vi "runtest update field value.vi"(1 "Process SPARTAN SN (F)":bool, 4 "ProcessNextItem? (f)":bool, 6 "User/Station":T1, 7 "POST (empty)":T4, 8 "error in (no error)":errorcluster, 9 "Model Number (\"\")":string, 10 "Field":T6={"ixField"=0, "iSequenceOrder"=0, "sxFieldId"="", "sxSequenceId"="", "sDisplayName"="", "sValue"="", "sUnits"="", "nDataType"=enum."timestamp", "nNextItem"=enum."Reset", "fSystem"=FALSE, "fSystemValue"=FALSE, "fRequired"=FALSE, "fSetAtTest"=FALSE, "fTestField"=FALSE, "fDeleted"=FALSE, "fIndexed"=FALSE, "fFreeList"=FALSE}, 11 "Connection Refnum":T5) -> (0 "error out":errorcluster, 2 "updated Field":T6={"ixField"=0, "iSequenceOrder"=0, "sxFieldId"="", "sxSequenceId"="", "sDisplayName"="", "sValue"="", "sUnits"="", "nDataType"=enum."timestamp", "nNextItem"=enum."Reset", "fSystem"=FALSE, "fSystemValue"=FALSE, "fRequired"=FALSE, "fSetAtTest"=FALSE, "fTestField"=FALSE, "fDeleted"=FALSE, "fIndexed"=FALSE, "fFreeList"=FALSE}, 3 "Connection Refnum":T5, 5 "remaining POST":T4)   [LabVIEW 2011]
uses:
  server/database/Fields/Field Record.ctl
  server/database/Fields/Field DataTypes.ctl
  server/database/Fields/Field NextItem.ctl
  Addons/internet/utils/keyedarr.llb/Keyed Array.ctl
  SI.LIB/ODBC/SQL Controls/Connection Refnum.ctl
  runtest User - Station.ctl
  server/database/Stations/Instruments/Instrument Record.ctl
  server/database/Stations/Step Associations/Step Association Record.ctl
  Addons/internet/utils/strutil.llb/Case Matching.ctl
  server/server lib/Spartan Version.vi
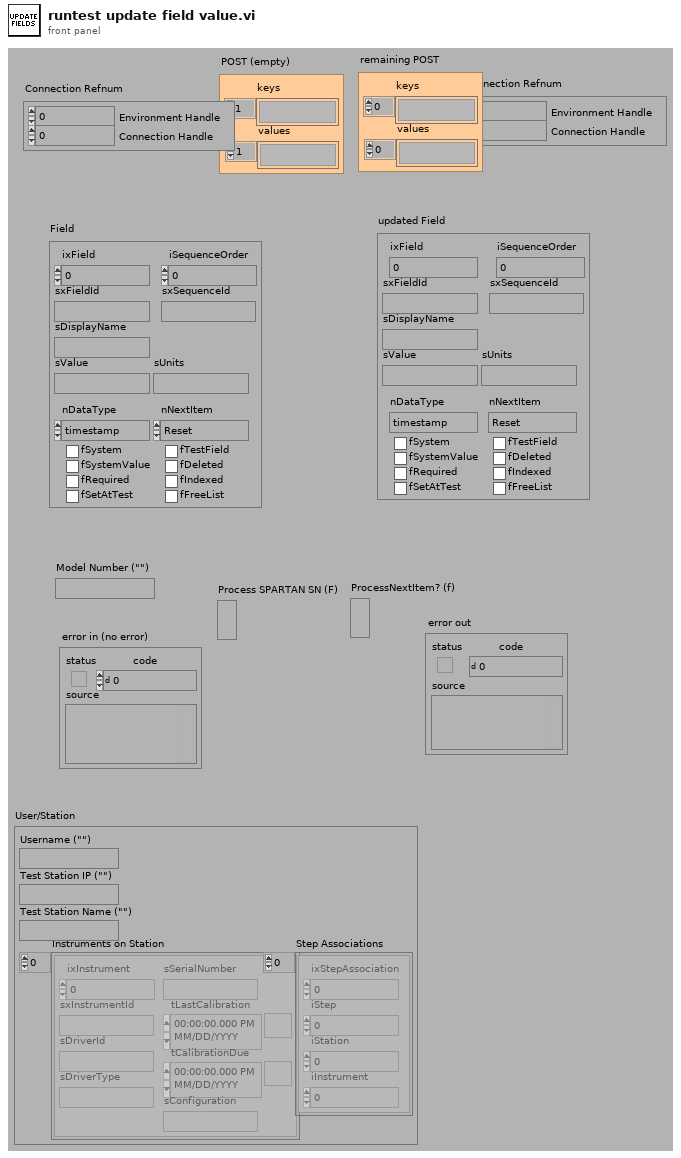
[diagram p1: front panel]
types:
  T1 = typedef "runtest User - Station.ctl" = cluster{"Username (\"\")":string, "Test Station IP (\"\")":string, "Test Station Name (\"\")":string, "Instruments on Station":T2[], "Step Associations":T3[]}
  T2 = typedef "Instrument Record.ctl" = cluster{"ixInstrument":i32, "sxInstrumentId":string, "sDriverId":string, "sDriverType":string, "sSerialNumber":string, "tLastCalibration":timestamp, "tCalibrationDue":timestamp, "sConfiguration":string}
  T3 = typedef "Step Association Record.ctl" = cluster{"ixStepAssociation":i32, "iStep":i32, "iStation":i32, "iInstrument":i32}
  T4 = typedef "Keyed Array.ctl" = cluster{"keys":string[], "values":string[]}
  T5 = typedef "Connection Refnum.ctl" = cluster{"Environment Handle":i32, "Connection Handle":i32}
  T6 = typedef "Field Record.ctl" = cluster{"ixField":i32, "iSequenceOrder":i32, "sxFieldId":string, "sxSequenceId":string, "sDisplayName":string, "sValue":string, "sUnits":string, "nDataType":T7, "nNextItem":T8, "fSystem":bool, "fSystemValue":bool, "fRequired":bool, "fSetAtTest":bool, "fTestField":bool, "fDeleted":bool, "fIndexed":bool, "fFreeList":bool}
  T7 = typedef "Field DataTypes.ctl" = enum32{"text", "numeric", "list", "timestamp", "boolean"}
  T8 = typedef "Field NextItem.ctl" = enum32{"Reset", "Retain", "Auto-Increment"}
  T9 = typedef "Case Matching.ctl" = enum16{"a != A", "a == A", "system"}
  T10 = typedef "OGAB Version.ctl" = cluster{"Version":string, "Build Number":u32, "Build Date/Time":dbl}
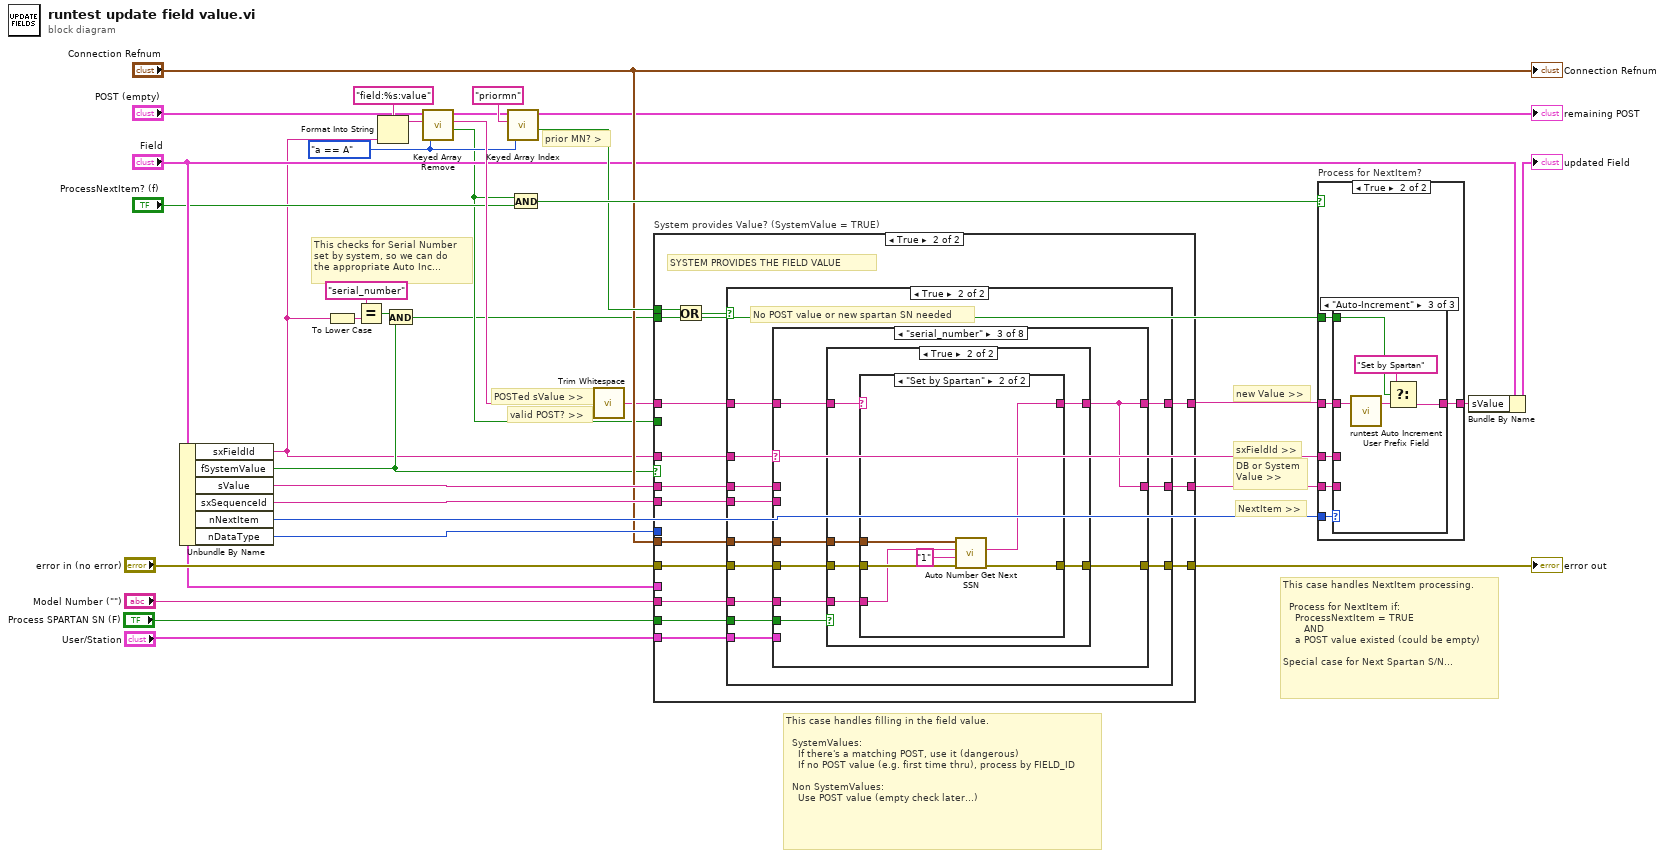
[diagram p0: block diagram]
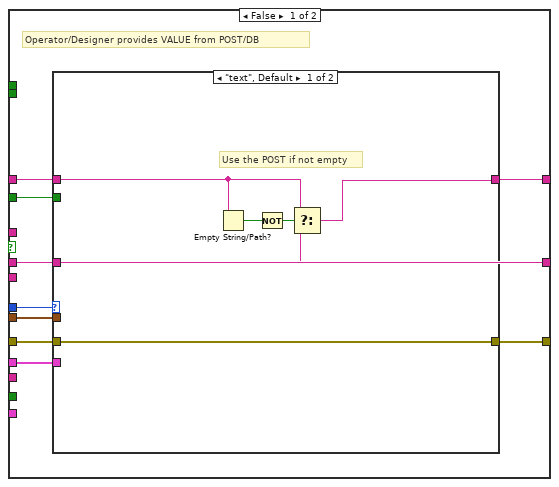
[diagram p5: hidden frame]
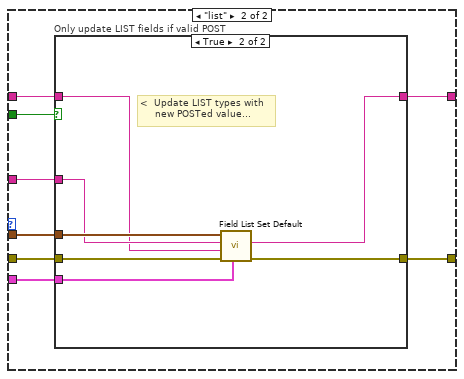
[diagram p6: hidden frame]
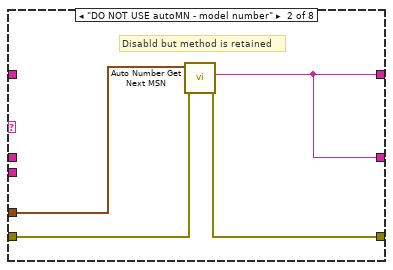
[diagram p10: hidden frame]
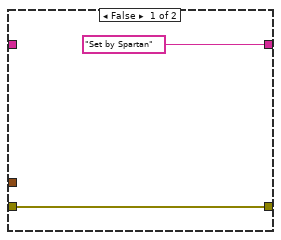
[diagram p11: hidden frame]
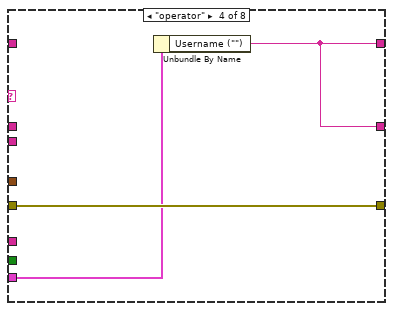
[diagram p13: hidden frame]
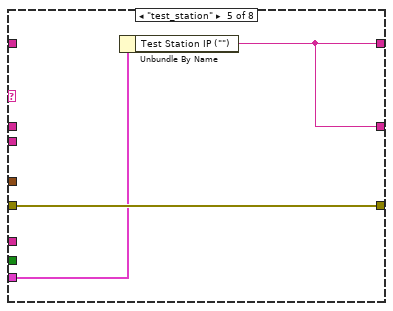
[diagram p14: hidden frame]
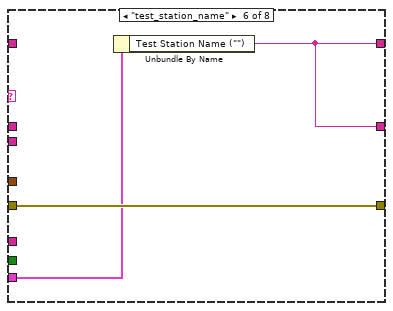
[diagram p15: hidden frame]
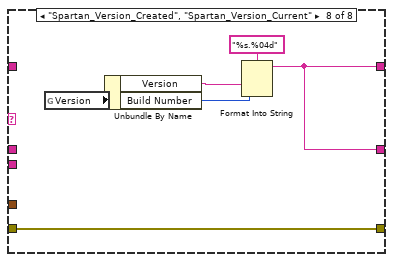
[diagram p17: hidden frame]
diagram:
  w10 = Case_Matching."a == A" ("case matching (sensitive)")
  # "sxFieldId >>"
  # "prior MN? >"
  # "POSTed sValue >>"
  # "This checks for Serial Number\nset by system, so we can do\nthe appropriate Auto Inc..."
  # "valid POST? >>"
  # "DB or System\nValue >>"
  # "new Value >>"
  # "NextItem >>"
  # "This case handles NextItem processing.\n\n  Process for NextItem if:\n    ProcessNextItem = TRUE\n       AND\n    a POST value existed (could be empty)\n\nSpecial case for Next Spartan S/N..."
  # "This case handles filling in the field value. \n\n  SystemValues:\n    If there's a matching POST, use it (dangerous)\n    If no POST value (e.g. first time thru), process by FIELD_ID\n\n  Non SystemValues:\n    Use POST value (empty check later...)"
  n1 = Unbundle By Name("Field") -> ("sxFieldId"=w5:string, "fSystemValue"=w9:bool, "sValue"=w23:string, "sxSequenceId"=w30:string, "nNextItem"=w26:T8, "nDataType"=w22:T7)
  n2 = To Lower Case(string=w5) -> (all lower case string=w8:string)
  n3 = Equal?(x="serial_number" ("Field_ID"), y=w8) -> (x = y?=w6:bool)
  n4 = Format Into String(format string="field:%s:value", w5) -> (resulting string=w33:string)  [unwired: 2 in, 1 out]
  n5 = And(x=w6, y=w9) -> (x .and. y?=w2:bool)
  n6 = call "Keyed Array Remove.vi"("case matching (sensitive)"=w10, "key"=w33, "array in"="POST (empty)") -> ("valid key"=w4:bool, "value"=w32:string, "array out"=w12:T4)  [unwired: 2 out]
  n7 = call "Keyed Array Index.vi"("case matching (sensitive)"=w10, "key"="priormn", "array in"=w12) -> ("valid key"=w18:bool, "duplicate array"=→"remaining POST":T4)  [unwired: 1 in, 2 out]
  n8 = And(x=w4, y="ProcessNextItem? (f)") -> (x .and. y?=w27:bool)
  n9 = call <vilib>:"Trim Whitespace.vi"("string"=w32) -> ("trimmed string"=w1:string)  [unwired: 1 in]
  n10 = case "System provides Value? (SystemValue = TRUE)" shown="True" w9 {
    tunnel: "error in (no error)" -> [w40 w81]
    tunnel: w23 -> [w42 w76]
    tunnel: w1 -> [w41 w80]
    tunnel: [w39 w79] -> w3
    tunnel: [w43 w78] -> w29
    tunnel: w5 -> [_ w77]
    tunnel: "User/Station" -> [_ w75]
    tunnel: "Model Number (\"\")" -> [_ w70]
    tunnel: w30 -> [_ w74]
    tunnel: [w42 w73] -> w28
    tunnel: w22 -> [w36 _]
    tunnel: w2 -> [_ w68]
    tunnel: w18 -> [_ w69]
    tunnel: "Process SPARTAN SN (F)" -> [_ w72]
    tunnel: "Connection Refnum" -> [w38 w71]
    tunnel: "Field" -> [w37 _]
    tunnel: w4 -> [w35 _]
    frame False {
      # "Operator/Designer provides VALUE from POST/DB"
      n11 = case shown="\"text\", Default" w36 {
        tunnel: [w49 w53] -> w43
        tunnel: w42 -> [w47 w54]
        tunnel: w41 -> [w45 w52]
        tunnel: w40 -> [w46 w56]
        tunnel: [w46 w55] -> w39
        tunnel: w38 -> [_ w57]
        tunnel: w37 -> [_ w51]
        tunnel: w35 -> [_ w50]
        frame "text", Default {
          # "Use the POST if not empty"
          n12 = Empty String/Path?(string/path=w45) -> (empty?=w44:bool)
          n13 = Not(x=w44) -> (.not. x?=w48:bool)
          n14 = Select(t=w45, s=w48, f=w47) -> (s? t:f=w49:string)
        }
        frame "list" {
          n15 = case "Only update LIST fields if valid POST" shown="True" w50 {
            tunnel: w57 -> [_ w66]
            tunnel: w56 -> [w58 w65]
            tunnel: [w58 w64] -> w55
            tunnel: w54 -> [w59 w63]
            tunnel: [w59 w62] -> w53
            tunnel: w52 -> [_ w61]
            tunnel: w51 -> [_ w60]
            frame False {
              # "< NOT a valid POSTed sValue\n    Leave the LIST item as is from DB"
            }
            frame True {
              # "<  Update LIST types with\n     new POSTed value..."
              n16 = call "Field List Set Default.vi"("FIELD (empty)"=w60, "error in (no error)"=w65, "Default Value (\"\")"=w61, "Flat List (\"\")"=w63, "Connection Refnum"=w66) -> ("error out"=w64:errorcluster, "New Flat List"=w62:string)  [unwired: 5 out]
            }
          }
        }
      }
    }
    frame True {
      # "SYSTEM PROVIDES THE FIELD VALUE"
      n17 = Or(x=w69, y=w68) -> (x .or. y?=w67:bool)
      n18 = case shown="True" w67 {
        tunnel: w81 -> [w83 w95]
        tunnel: w80 -> [w82 w91]
        tunnel: [w82 w94] -> w78
        tunnel: [w83 w93] -> w79
        tunnel: w77 -> [_ w92]
        tunnel: w76 -> [_ w90]
        tunnel: w75 -> [_ w89]
        tunnel: w74 -> [_ w88]
        tunnel: [w82 w87] -> w73
        tunnel: w72 -> [_ w86]
        tunnel: w70 -> [_ w85]
        tunnel: w71 -> [_ w84]
        frame False {
          # "Not serial_number OR priorMN"
        }
        frame True {
          # "No POST value or new spartan SN needed"
          n19 = case shown="\"serial_number\"" w92 {
            tunnel: w95 -> [w97 w101 w108 w127 w130 w133 w135 w141]
            tunnel: [w96 w99 w105 w125 w128 w131 w134 w136] -> w94
            tunnel: [w97 w100 w107 w127 w130 w133 w135 w141] -> w93
            tunnel: w91 -> [_ _ w102 _ _ _ _ _]
            tunnel: w90 -> [w96 _ _ _ _ _ _ _]
            tunnel: w89 -> [_ _ _ w126 w129 w132 _ _]
            tunnel: w88 -> [_ _ _ _ _ _ w134 _]
            tunnel: [w96 w99 w105 w125 w128 w131 w134 w136] -> w87
            tunnel: w86 -> [_ _ w106 _ _ _ _ _]
            tunnel: w85 -> [_ _ w104 _ _ _ _ _]
            tunnel: w84 -> [_ w98 w103 _ _ _ _ _]
            frame "UNKNOWN", Default {
            }
            frame "DO NOT USE autoMN - model number" {
              # "Disabld but method is retained"
              n20 = call "Auto Number Get Next MSN.vi"("error in (no error)"=w101, "Connection Refnum"=w98) -> ("error out"=w100:errorcluster, "Model Number"=w99:string)  [unwired: 8 out]
            }
            frame "serial_number" {
              n21 = case shown="True" w106 {
                tunnel: w108 -> [w109 w116]
                tunnel: [w109 w115] -> w107
                tunnel: ["Set by Spartan" ("key") w112] -> w105
                tunnel: w104 -> [_ w114]
                tunnel: w103 -> [_ w113]
                tunnel: w102 -> [_ w111]
                frame False {
                }
                frame True {
                  n22 = case shown="\"Set by Spartan\"" w111 {
                    selector: w111 -> [w117 _]
                    tunnel: w116 -> [w118 w124]
                    tunnel: [w118 w123] -> w115
                    tunnel: w114 -> [_ w122]
                    tunnel: w113 -> [_ w121]
                    tunnel: [w117 w120] -> w112
                    frame "NOP", Default {
                    }
                    frame "Set by Spartan" {
                      n23 = call "Auto Number Get Next SSN.vi"("error in (no error)"=w124, "Initial Serial Number (1)"="1", "Model Number"=w122, "Connection Refnum"=w121) -> ("error out"=w123:errorcluster, "Spartan Serial Number"=w120:string)  [unwired: 1 in, 5 out]
                    }
                  }
                }
              }
            }
            frame "operator" {
              n24 = Unbundle By Name(w126) -> ("Username (\"\")"=w125:string)
            }
            frame "test_station" {
              n25 = Unbundle By Name(w129) -> ("Test Station IP (\"\")"=w128:string)
            }
            frame "test_station_name" {
              n26 = Unbundle By Name(w132) -> ("Test Station Name (\"\")"=w131:string)
            }
            frame "test_sequence" {
            }
            frame "Spartan_Version_Created", "Spartan_Version_Current" {
              n27 = global read "Spartan Version.vi" "Version"() -> (w140:T10)
              n28 = Unbundle By Name(w140) -> ("Version"=w138:string, "Build Number"=w137:u32)
              n29 = Format Into String(format string="%s.%04d", w138, w137) -> (resulting string=w136:string)  [unwired: 2 in, 1 out]
            }
          }
        }
      }
    }
  }
  "error out" <- w3
  n30 = case "Process for NextItem?" shown="True" w27 {
    tunnel: w26 -> [_ w148]
    tunnel: w29 -> [w142 w147]
    tunnel: [w142 w145] -> w20
    tunnel: w28 -> [_ w146]
    tunnel: w5 -> [_ w144]
    tunnel: w2 -> [_ w143]
    frame False {
    }
    frame True {
      n31 = case shown="\"Auto-Increment\"" w148 {
        tunnel: w147 -> [_ w150 w152]
        tunnel: [w149 w150 w151] -> w145
        tunnel: w146 -> [w149 _ _]
        tunnel: w144 -> [_ _ _]
        tunnel: w143 -> [_ _ w155]
        frame "Reset", Default {
        }
        frame "Retain" {
        }
        frame "Auto-Increment" {
          n32 = call "runtest Auto Increment User Prefix Field.vi"("Field Value"=w152) -> ("New Field Value"=w153:string)  [unwired: 2 out]
          n33 = Select(t="Set by Spartan" ("key"), s=w155, f=w153) -> (s? t:f=w151:string)
        }
      }
    }
  }
  n34 = Bundle By Name(cluster="Field", "sValue"=w20) -> (→"updated Field":T6)
  "Connection Refnum" <- "Connection Refnum"
